vi "IDS_lock.vi"(8 "error in (no error)":errorcluster, 9 "password":string, 11 "deviceHandle":i32) -> (0 "error out":errorcluster, 3 "deviceHandle out":i32)   [LabVIEW 2016]
panel:
  out "password out":string
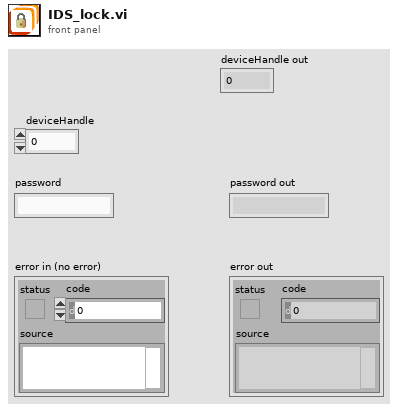
[diagram p1: front panel]
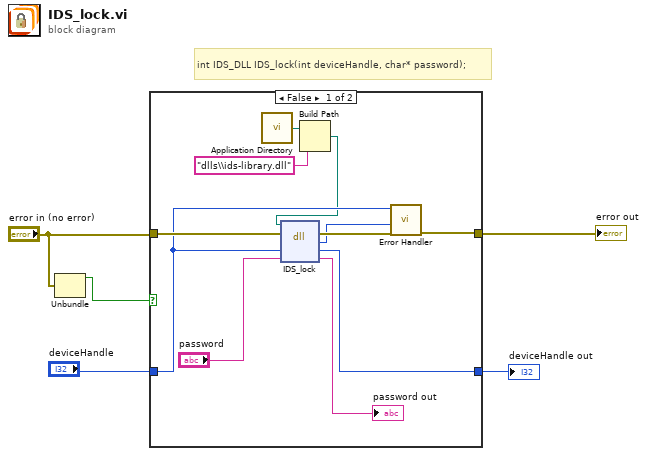
[diagram p0: block diagram]
diagram:
  # "int IDS_DLL IDS_lock(int deviceHandle, char* password);"
  n1 = Unbundle("error in (no error)") -> ("status"=w1:bool)  [unwired: 2 out]
  n2 = case shown="False" w1 {
    tunnel: "error in (no error)" -> [w14 w18]
    tunnel: [w11 w18] -> w5
    tunnel: "deviceHandle" -> [w9 w17]
    tunnel: [w13 w17] -> w3
    frame False {
      n3 = call <vilib>:"Application Directory.vi"() -> ("Application Directory"=w8:path)
      n4 = Build Path(base path=w8, name or relative path="dlls\\ids-library.dll" ("ipAddress")) -> (appended path=w6:path)
      n5 = dll-call lib="C:/Users/matheus/Desktop/LabVIEW_Draft_V1.6.0/dlls/ids-library.*" fn="IDS_lock"(path in=w6, error in=w14, "deviceHandle"=w9, "password"="password") -> (error out=w12:errorcluster, "return type"=w10:i32, "deviceHandle"=w13:i32, "password"=→"password out":string)  [unwired: 1 in, 1 out]
      n6 = call "Error Handler.vi"("error in (no error)"=w12, "error code"=w10, "deviceHandle"=w9) -> ("error out"=w11:errorcluster)  [unwired: 7 in, 1 out]
    }
    frame True {
    }
  }
  "error out" <- w5
  "deviceHandle out" <- w3
